vi "Design Challenge 1.vi"() -> ()   [LabVIEW 2019]
panel:
  in  "?":bool
  in  "?":bool
  out "Height (m)":dbl
  out "Distance (m)":dbl
  out "Trajectory":cluster{dbl[], dbl[]}[](graph)
  in  "Launch Angle (deg)":dbl min=0.0 max=89.0
  in  "Initial Velocity (m/s)":dbl min=0.0
  in  "Initial Height (m)":dbl min=0.0
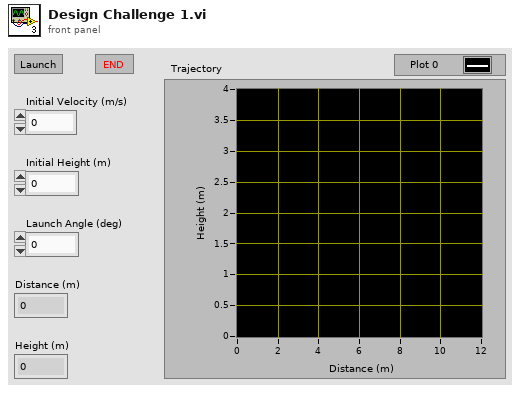
[diagram p1: front panel]
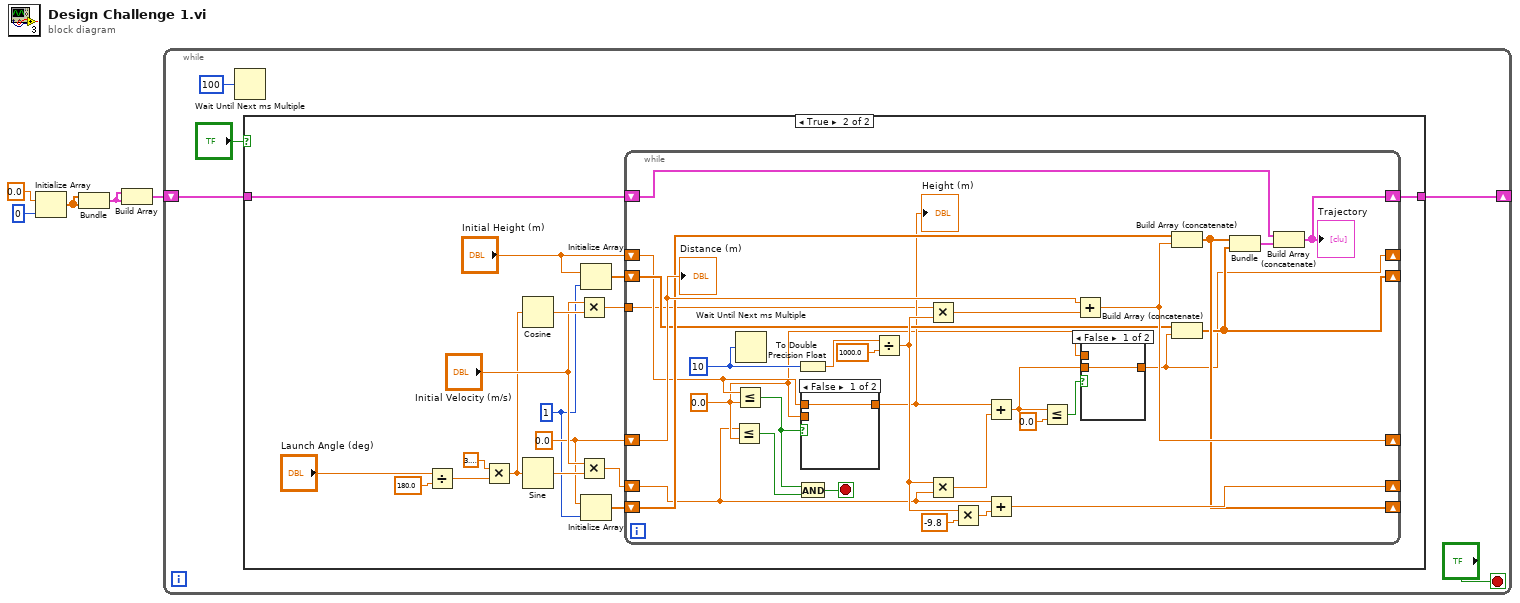
[diagram p0: block diagram]
diagram:
  n1 = Initialize Array(0.0 ("element"), 0 ("dimension size")) -> (w3:dbl[])
  n2 = Bundle(w3, w3) -> (w1:cluster{dbl[], dbl[]})  [unwired: 1 in]
  n3 = Build Array(w1, w1) -> (w2:cluster{dbl[], dbl[]}[])
  n4 = while {
    shift-right: [w7] -> _
    shift-left: w2 -> [w6]
    stop <- "?" stop-if-true
    n5 = Wait Until Next ms Multiple(millisecond multiple=u32 100) -> ()  [unwired: 1 out]
    n6 = case shown="True" "?" {
      tunnel: [w11 w13] -> w7
      tunnel: w6 -> [w11 w12]
      frame False {
      }
      frame True {
        w21 = 1
        w23 = 0.0
        n7 = Divide(x="Launch Angle (deg)", y=180.0) -> (x/y=w15:dbl)
        n8 = Multiply(x=3.141592653589793, y=w15) -> (x*y=w14:dbl)
        n9 = Cosine(x=w14) -> (cos(x)=w28:dbl)
        n10 = Sine(x=w14) -> (sin(x)=w27:dbl)
        n11 = Multiply(x="Initial Velocity (m/s)", y=w28) -> (x*y=w24:dbl)
        n12 = Multiply(x="Initial Velocity (m/s)", y=w27) -> (x*y=w25:dbl)
        n13 = Initialize Array("Initial Height (m)", w21) -> (w19:dbl[])
        n14 = Initialize Array(w23, w21) -> (w20:dbl[])
        n15 = while {
          shift-right: [w48] -> _
          shift-left: w23 -> [w54]
          shift-right: [w38] -> _
          shift-left: "Initial Height (m)" -> [w40]
          shift-right: [w49] -> _
          shift-left: w25 -> [w29]
          tunnel: w24 -> [w30]
          shift-right: [w44] -> _
          shift-left: w19 -> [w45]
          shift-right: [w46] -> _
          shift-left: w20 -> [w47]
          shift-right: [w43] -> w13
          shift-left: w12 -> [w41]
          stop <- w33 stop-if-true
          w31 = 0.0
          w57 = u32 10 ("millisecond multiple")
          n16 = Less Or Equal?(x=w29, y=w31) -> (x <= y?=w32:bool)
          n17 = Less Or Equal?(x=w40, y=w31) -> (x <= y?=w34:bool)
          n18 = Wait Until Next ms Multiple(millisecond multiple=w57) -> ()  [unwired: 1 out]
          n19 = To Double Precision Float(number=w57) -> (double precision float=w56:dbl)
          n20 = And(x=w34, y=w32) -> (x .and. y?=w33:bool)
          n21 = case shown="False" w34 {
            tunnel: [w61 w62] -> w39
            tunnel: w31 -> [_ w62]
            tunnel: w40 -> [w61 _]
            frame False {
            }
            frame True {
            }
          }
          "Height (m)" <- w39
          n22 = Divide(x=w56, y=1000.0) -> (x/y=w52:dbl)
          n23 = Multiply(x=w30, y=w52) -> (x*y=w55:dbl)
          n24 = Multiply(x=w52, y=w29) -> (x*y=w53:dbl)
          n25 = Multiply(x=w52, y=-9.8) -> (x*y=w50:dbl)
          n26 = Add(x=w39, y=w53) -> (x+y=w36:dbl)
          n27 = Add(x=w29, y=w50) -> (x+y=w49:dbl)
          n28 = Less Or Equal?(x=w36, y=0.0) -> (x <= y?=w35:bool)
          n29 = Add(x=w54, y=w55) -> (x+y=w48:dbl)
          n30 = case shown="False" w35 {
            tunnel: [w59 w60] -> w38
            tunnel: w31 -> [_ w60]
            tunnel: w36 -> [w59 _]
            frame False {
            }
            frame True {
            }
          }
          n31 = Build Array (concatenate)(w47, w48) -> (w46:dbl[])
          n32 = Build Array (concatenate)(w45, w38) -> (w44:dbl[])
          n33 = Bundle(w46, w44) -> (w42:cluster{dbl[], dbl[]})  [unwired: 1 in]
          n34 = Build Array (concatenate)(w41, w42) -> (w43:cluster{dbl[], dbl[]}[])
          "Trajectory" <- w43
          "Distance (m)" <- w54
        }
      }
    }
  }
